vi "PH_GUI.set I16 ring GUI object.vi"(2 "Ring Ref":refnum<vi>, 3 "Value":i16, 4 "Blinking (false)":bool, 5 "error in (no error)":errorcluster, 7 "Tip Strip":string="N/A") -> (19 "error out":errorcluster)   [LabVIEW 2014, in "PH_Common.lvlib"]
doc: "Sets value and more for the referenced GUI object."
uses:
  PH_Common.lvlib
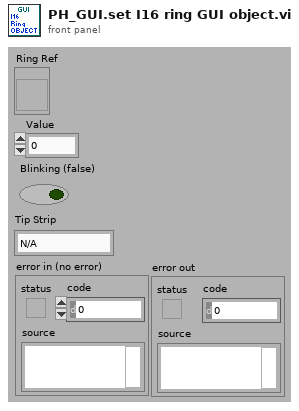
[diagram p1: front panel]
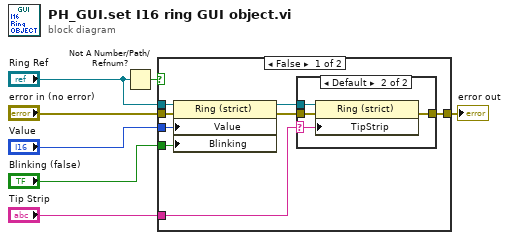
[diagram p0: block diagram]
diagram:
  n1 = Not A Number/Path/Refnum?(number/path/refnum="Ring Ref") -> (NaN/Path/Refnum?=w4:bool)
  n2 = case shown="False" w4 {
    tunnel: "error in (no error)" -> [w15 w21]
    tunnel: [w10 w21] -> w5
    tunnel: "Ring Ref" -> [w14 _]
    tunnel: "Value" -> [w13 _]
    tunnel: "Blinking (false)" -> [w12 _]
    tunnel: "Tip Strip" -> [w8 _]
    frame False {
      n3 = property class="Ring (strict)"(reference=w14, error in=w15, "Value"=w13, "Blinking"=w12) -> (reference out=w9:refnum<vi>, error out=w11:errorcluster)
      n4 = case shown="Default" w8 {
        selector: w8 -> [_ w17]
        tunnel: w11 -> [w16 w20]
        tunnel: [w16 w19] -> w10
        tunnel: w9 -> [_ w18]
        frame "", "N/A" {
        }
        frame Default {
          n5 = property class="Ring (strict)"(reference=w18, error in=w20, "TipStrip"=w17) -> (error out=w19:errorcluster)  [unwired: 1 out]
        }
      }
    }
    frame True {
    }
  }
  "error out" <- w5
